vi "sv_Insert Swept FRF Values.vi"(8 "scaled measurements in":T1 {"harmonic components [ratio]" format="%.2f"; "THD [ratio]" format="%.2f"; "FRF Measurements"."Im [response]" format="%.2f"; "FRF Measurements"."Re [response]" format="%.2f"; "FRF Measurements"."Im [stimulus]" format="%.2f"; "FRF Measurements"."Re [stimulus]" format="%.2f"; "RMS response" format="%.2f"; "RMS stimulus" format="%.2f"}, 10 "AI freq index":i32, 11 "measurements in":T2 {"scaled response magnitude" format="%.3f"; "Harm[]" format="%.2f"; "THD" format="%.2f"; "Im [response]" format="%.2f"; "Re [response]" format="%.2f"; "Im [stimulus]" format="%.2f"; "Re [stimulus]" format="%.2f"; "RMS response" format="%.2f"; "RMS stimulus" format="%.2f"}) -> (0 "dup new measurements":T1 {"harmonic components [ratio]" format="%.2f"; "THD [ratio]" format="%.2f"; "FRF Measurements"."Im [response]" format="%.2f"; "FRF Measurements"."Re [response]" format="%.2f"; "FRF Measurements"."Im [stimulus]" format="%.2f"; "FRF Measurements"."Re [stimulus]" format="%.2f"; "RMS response" format="%.2f"; "RMS stimulus" format="%.2f"}, 2 "dup AI freq index":i32, 3 "measurements in":T2 {"scaled response magnitude" format="%.3f"; "Harm[]" format="%.2f"; "THD" format="%.2f"; "Im [response]" format="%.2f"; "Re [response]" format="%.2f"; "Im [stimulus]" format="%.2f"; "Re [stimulus]" format="%.2f"; "RMS response" format="%.2f"; "RMS stimulus" format="%.2f"})   [LabVIEW 2017, in "SoundVib_SweptSine.lvlib"]
uses:
  <vilib>/addons/Sound and Vibration/svt_Swept Sine/SoundVib_SweptSine.lvlib
  <vilib>/addons/Sound and Vibration/svt_Swept Sine/subVIs/sv_Swept Sine Measurements.ctl
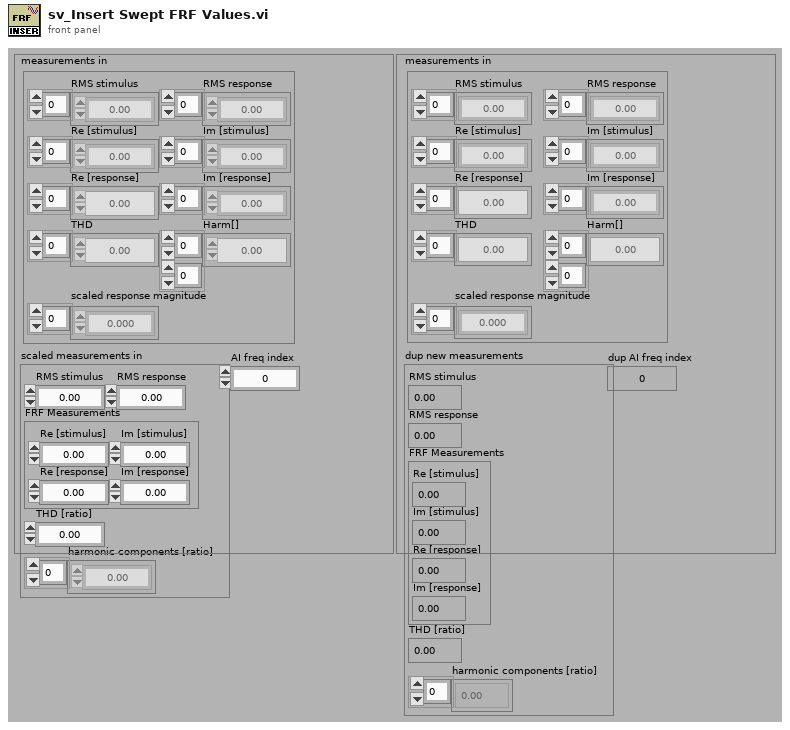
[diagram p1: front panel]
types:
  T1 = cluster{"RMS stimulus":dbl, "RMS response":dbl, "FRF Measurements":cluster{"Re [stimulus]":dbl, "Im [stimulus]":dbl, "Re [response]":dbl, "Im [response]":dbl}, "THD [ratio]":dbl, "harmonic components [ratio]":dbl[]}
  T2 = typedef "SoundVib_SweptSine.lvlib/sv_Swept Sine Measurements.ctl" = cluster{"RMS stimulus":dbl[], "RMS response":dbl[], "Re [stimulus]":dbl[], "Im [stimulus]":dbl[], "Re [response]":dbl[], "Im [response]":dbl[], "THD":dbl[], "Harm[]":dbl[][], "scaled response magnitude":dbl[]}
  T3 = cluster{"Re [stimulus]":dbl, "Im [stimulus]":dbl, "Re [response]":dbl, "Im [response]":dbl}
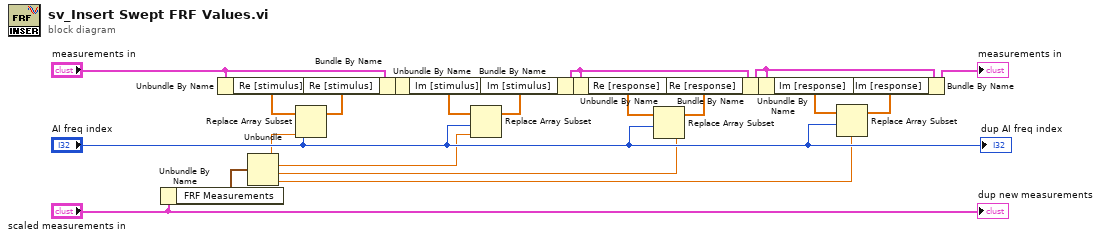
[diagram p0: block diagram]
diagram:
  n1 = Unbundle By Name("scaled measurements in") -> ("FRF Measurements"=w9:T3)
  n2 = Unbundle By Name("measurements in") -> ("Re [stimulus]"=w10:dbl[])
  n3 = Unbundle(w9) -> ("Re [stimulus]"=w11:dbl, "Im [stimulus]"=w16:dbl, "Re [response]"=w6:dbl, "Im [response]"=w3:dbl)
  n4 = Replace Array Subset(array=w10, new element=w11, index="AI freq index") -> (w12:dbl[])
  n5 = Bundle By Name(cluster="measurements in", "Re [stimulus]"=w12) -> (w14:T2)
  n6 = Unbundle By Name(w14) -> ("Im [stimulus]"=w13:dbl[])
  n7 = Replace Array Subset(array=w13, new element=w16, index="AI freq index") -> (w15:dbl[])
  n8 = Bundle By Name(cluster=w14, "Im [stimulus]"=w15) -> (w2:T2)
  n9 = Unbundle By Name(w2) -> ("Re [response]"=w8:dbl[])
  n10 = Replace Array Subset(array=w8, new element=w6, index="AI freq index") -> (w7:dbl[])
  n11 = Bundle By Name(cluster=w2, "Re [response]"=w7) -> (w1:T2)
  n12 = Unbundle By Name(w1) -> ("Im [response]"=w5:dbl[])
  n13 = Replace Array Subset(array=w5, new element=w3, index="AI freq index") -> (w4:dbl[])
  n14 = Bundle By Name(cluster=w1, "Im [response]"=w4) -> (→"measurements in":T2)
  "dup new measurements" <- "scaled measurements in"
  "dup AI freq index" <- "AI freq index"
